vi "open.vi"(8 "error in (no error)":errorcluster, 11 "K2602 in":refnum<class "K2602.lvclass">) -> (0 "error out":errorcluster, 3 "K2602 out":refnum<class "K2602.lvclass">)   [LabVIEW 2011, in "Hardware.lvlib" / "Channels.lvlib" / "K2602.lvclass"]
uses:
  K2602.lvclass
  K2602.lvclass/K2602.ctl
  <instrlib>/Keithley 2600 Series/Keithley 2600 Series.lvlib
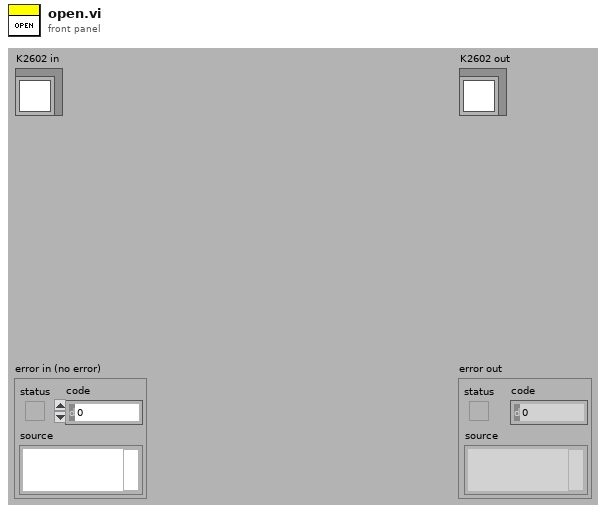
[diagram p1: front panel]
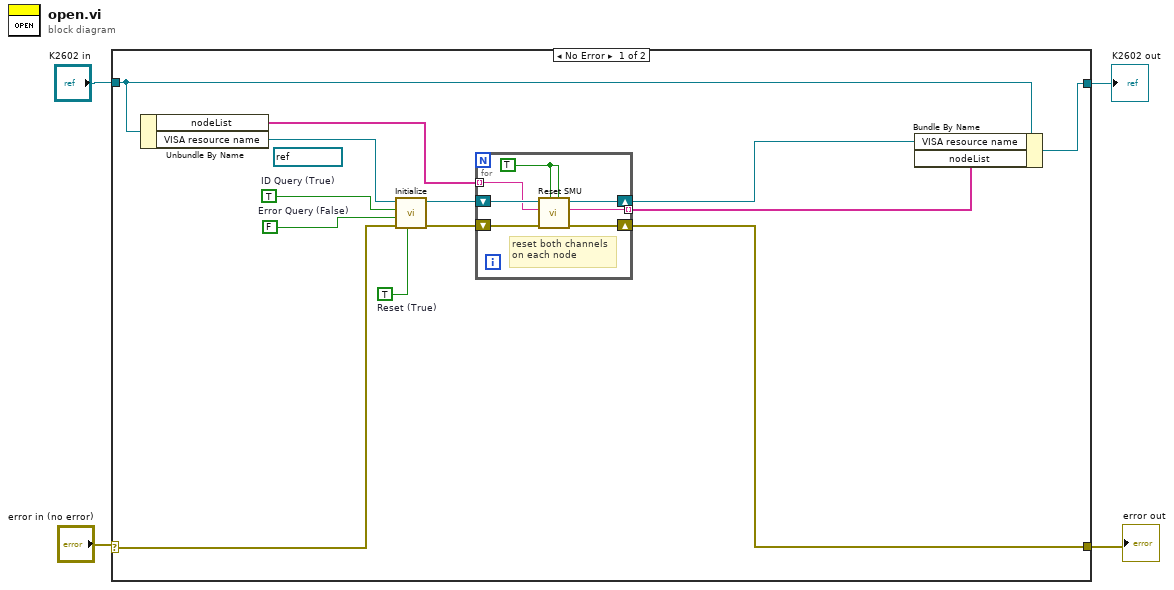
[diagram p0: block diagram]
diagram:
  n1 = case shown="No Error" "error in (no error)" {
    selector: "error in (no error)" -> [w14 w25]
    tunnel: [w16 w26] -> w3
    tunnel: "K2602 in" -> [w17 w26]
    tunnel: [w13 w25] -> w1
    frame No Error {
      w9 = FALSE  # Error Query (False)
      w10 = TRUE  # Reset (True)
      w12 = TRUE  # ID Query (True)
      (unwired) refnum<visa-resource-name> "keithley" ("VISA resource name")
      n2 = Unbundle By Name(w17) -> ("nodeList"=w7:string[], "VISA resource name"=w5:refnum<visa-resource-name>)
      n3 = call <instrlib>:"Initialize.vi"("Reset (True)"=w10, "error in (no error)"=w14, "Error Query (False)"=w9, "ID Query (True)"=w12, "VISA resource name"=w5) -> ("error out"=w8:errorcluster, "VISA resource name out"=w11:refnum<visa-resource-name>)  [unwired: 1 in, 4 out]
      n4 = for {
        tunnel: [w23] -> w6 mode=indexing
        shift-right: [w24] -> w15
        shift-left: w11 -> [w21]
        shift-right: [w22] -> w13
        shift-left: w8 -> [w19]
        tunnel: w7 -> [w18] mode=indexing
        w20 = TRUE
        # "reset both channels\non each node"
        n5 = call <instrlib>:"Reset SMU.vi"("SMU B (No)"=w20, "SMU A (No)"=w20, "error in (no error)"=w19, "Node In"=w18, "VISA resource name"=w21) -> ("error out"=w22:errorcluster, "Node Out"=w23:string, "VISA resource name out"=w24:refnum<visa-resource-name>)  [unwired: 4 out]
      }
      n6 = Bundle By Name(cluster=w17, "VISA resource name"=w15, "nodeList"=w6) -> (w16:refnum<class "K2602.lvclass">)
    }
    frame Error {
    }
  }
  "error out" <- w1
  "K2602 out" <- w3
